vi "1D I64.vi"(5 "format string (%.;%_20d)":string="%.;%_20d", 6 "collumn vector (F)":bool, 7 "key description":string, 8 "sections":string[](array[string]), 9 "numeric":i64[](array[numeric]), 11 "info data":string) -> (0 "sections out":string[](array[string]), 3 "info data out":string)   [LabVIEW 2020, in "infolib.lvlib"]
doc: "Add a new numeric table to Info Data string. If section exists in Info Data string, inserts key into this section. If collumn vector is set to false, the result will be one long line."
uses:
  infolib.lvlib
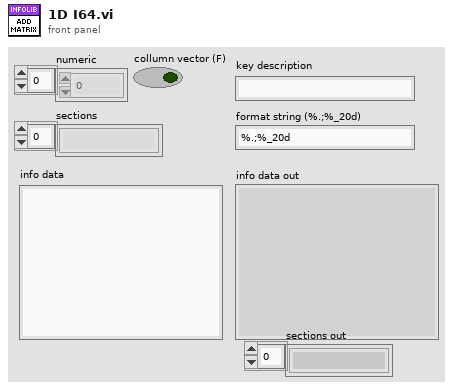
[diagram p1: front panel]
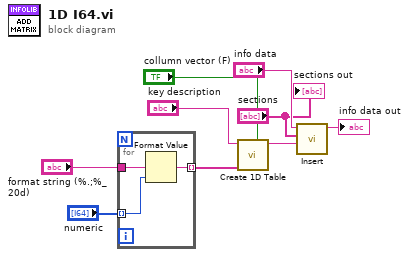
[diagram p0: block diagram]
diagram:
  n1 = for {
    tunnel: "numeric" -> [w12] mode=indexing
    tunnel: "format string (%.;%_20d)" -> [w11]
    tunnel: [w10] -> w3 mode=indexing
    n2 = Format Value(format string=w11, value (0)=w12) -> (output string=w10:string)  [unwired: 1 in]
  }
  n3 = call "Create 1D Table.vi"("collumn vector (F)"="collumn vector (F)", "formatted values"=w3, "table name"="key description") -> ("table"=w2:string)  [unwired: 7 in, 1 out]
  n4 = call "Insert.vi"("insert"=w2, "sections"="sections", "info data"="info data") -> ("info data out"=→"info data out":string)  [unwired: 8 in]
  "sections out" <- "sections"
